vi "AI Read.vi"() -> (0 "error":bool, 3 "waveforms":waveform(dbl)[](array[waveform]))   [LabVIEW 2023]
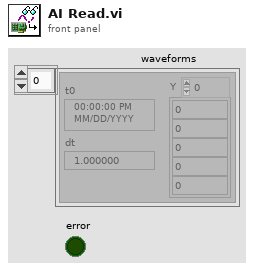
[diagram p1: front panel]
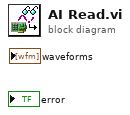
[diagram p0: block diagram]
diagram:
